vi "autophase.vi"(8 "error in (no error)":errorcluster, 11 "SR 830 & NI USB7855R in":refnum<class "SR 830 & NI USB7855R.lvclass">) -> (0 "error out":errorcluster, 3 "SR 830 & NI USB7855R out":refnum<class "SR 830 & NI USB7855R.lvclass">)   [LabVIEW 2020, in "SR 830 & NI USB7855R.lvclass"]
uses:
  SR 830 & NI USB7855R.lvclass
  SR 830 & NI USB7855R.lvclass/SR 830 & NI USB7855R.ctl
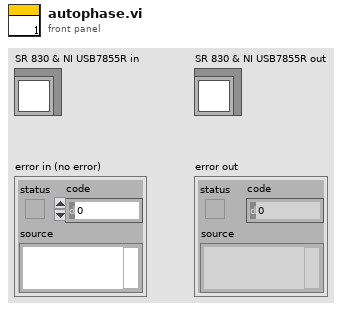
[diagram p1: front panel]
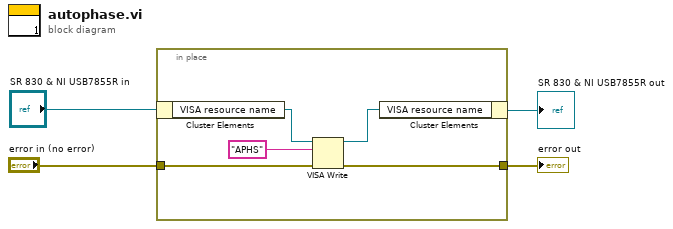
[diagram p0: block diagram]
diagram:
  n1 = in-place {
    in-place-border: "error in (no error)" -> [w8]
    in-place-border: [w6] -> w1
    n2 = in-place-cluster #1("SR 830 & NI USB7855R in") -> ("VISA resource name"=w9:refnum<visa-resource-name>)
    n3 = VISA Write(VISA resource name=w9, write buffer="APHS", error in (no error)=w8) -> (VISA resource name out=w5:refnum<visa-resource-name>, error out=w6:errorcluster)  [unwired: 1 out]
    n4 = in-place-cluster #1("VISA resource name"=w5) -> (→"SR 830 & NI USB7855R out":refnum<class "SR 830 & NI USB7855R.lvclass">)
  }
  "error out" <- w1
